vi "SetZoomMode.vi"(9 "Coords":T1, 10 "ZoomMode":refnum<vi>, 11 "XYGraph输入":refnum<vi>) -> ()   [LabVIEW 2015]
uses:
  <vilib>/Utility/miscctls.llb/LVPoint32TypeDef.ctl
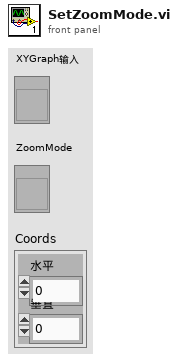
[diagram p1: front panel]
types:
  T1 = typedef "LVPoint32TypeDef.ctl" = cluster{"Horizontal":i32, "Vertical":i32}
  T2 = typedef "LVRectTypeDef.ctl" = cluster{"Left":i16, "Top":i16, "Right":i16, "Bottom":i16}
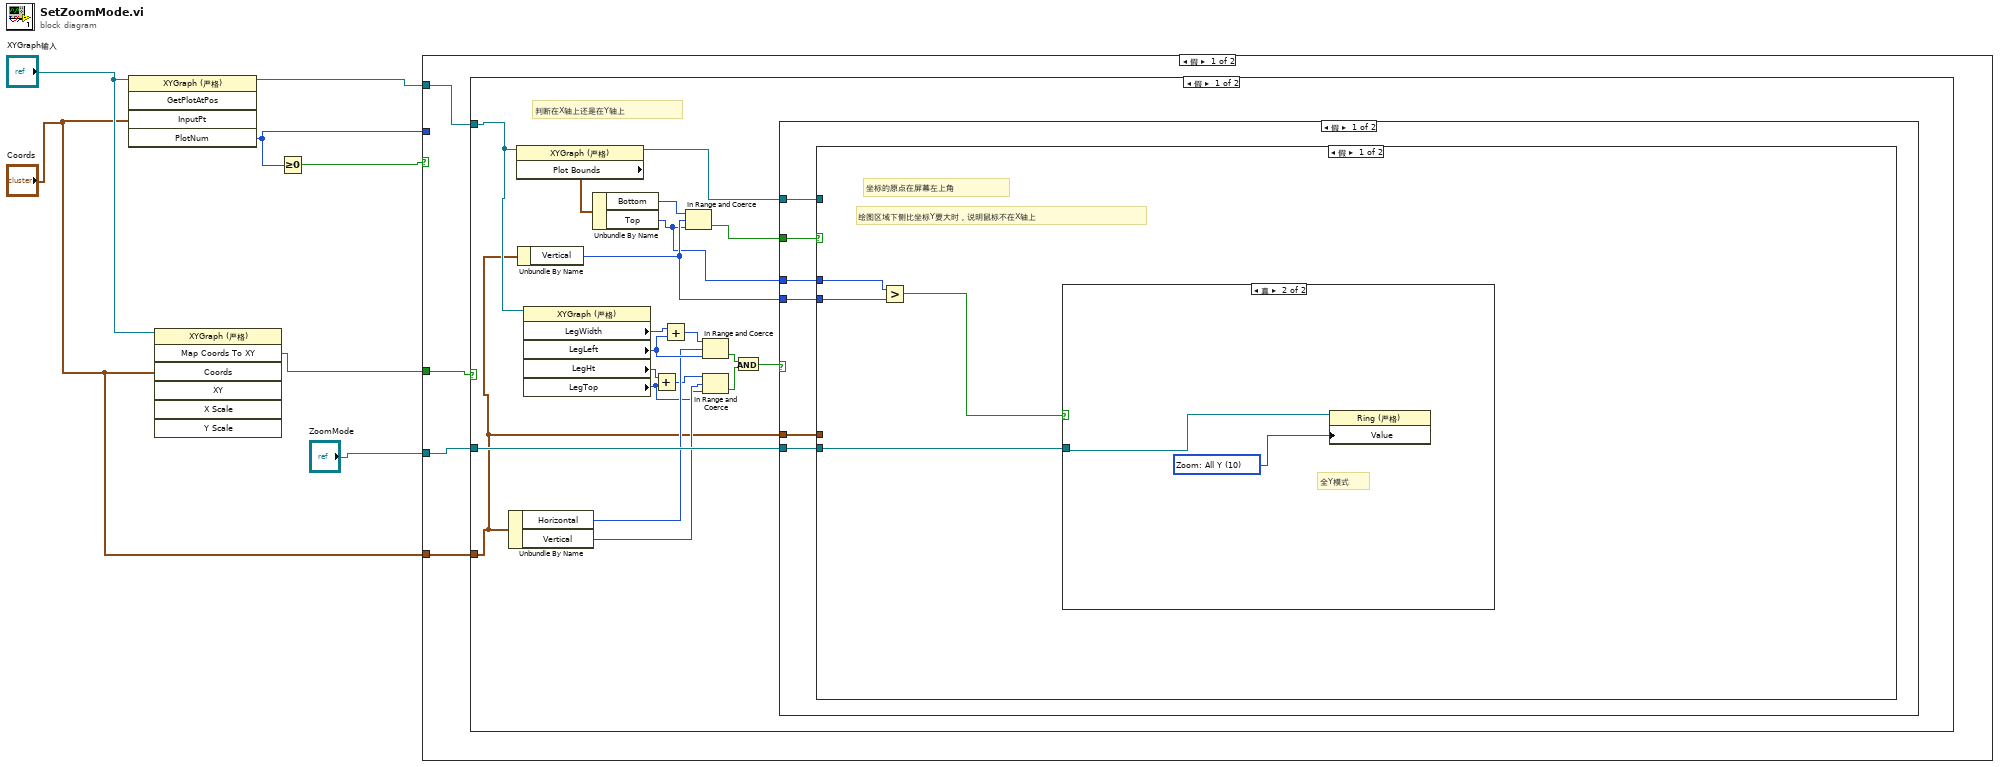
[diagram p0: block diagram]
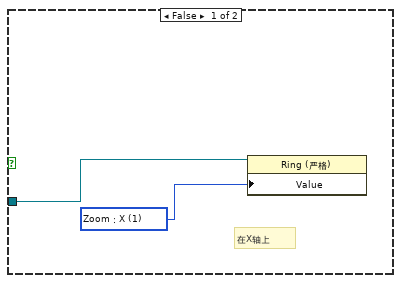
[diagram p2: hidden frame]
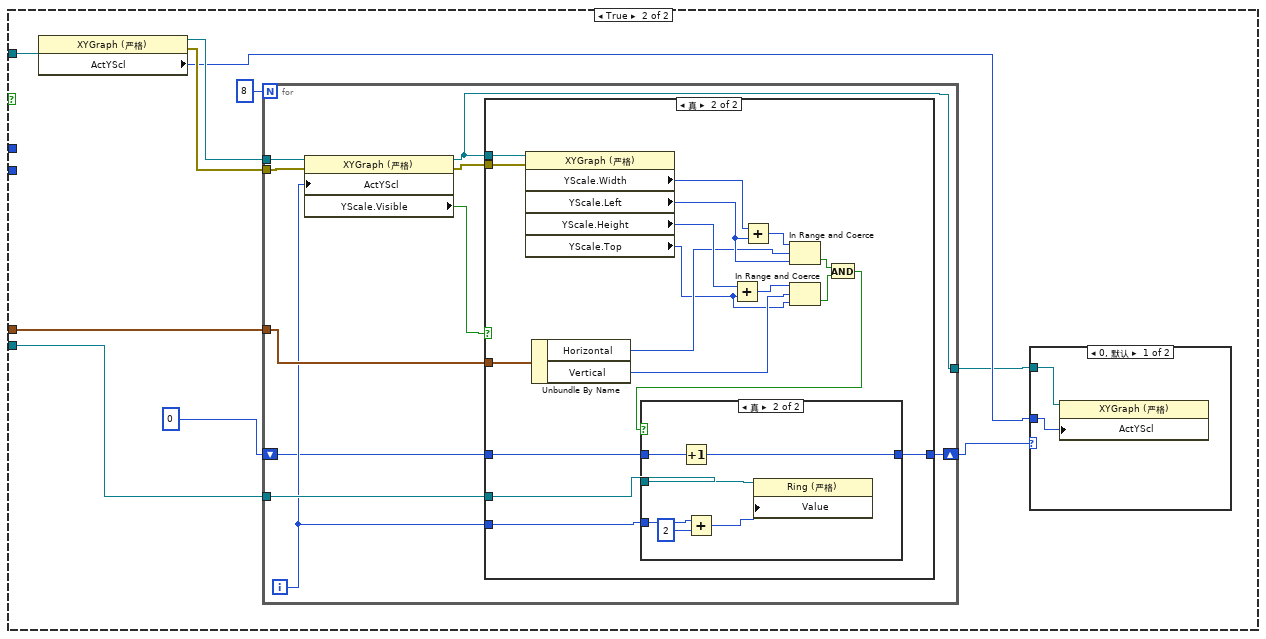
[diagram p3: hidden frame]
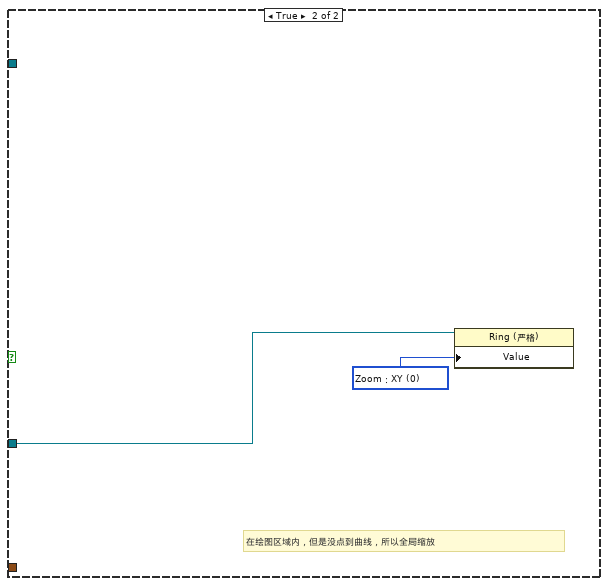
[diagram p8: hidden frame]
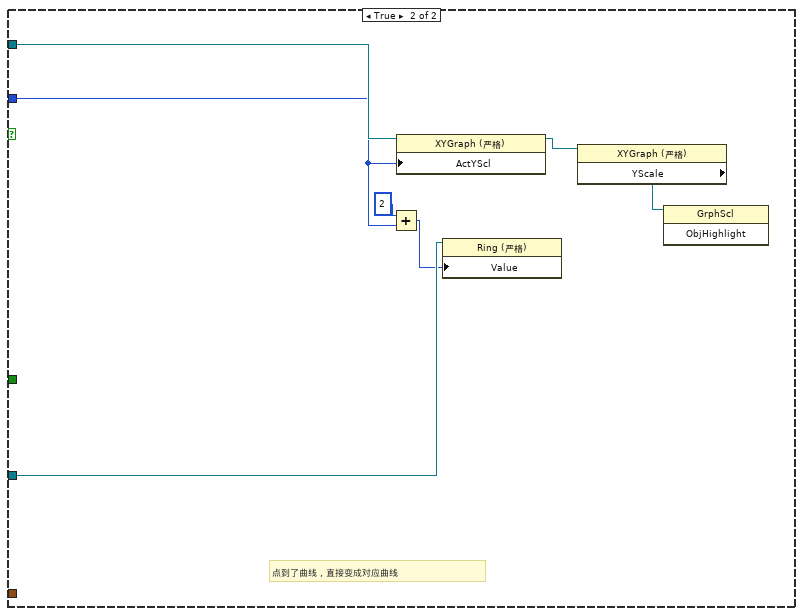
[diagram p9: hidden frame]
diagram:
  n1 = invoke class="XYGraph (严格)" method="GetPlotAtPos"(reference="XYGraph输入", "InputPt"="Coords") -> (reference out=w4:refnum<vi>, "PlotNum"=w3:i32)  [unwired: 3 in, 3 out]
  n2 = invoke class="XYGraph (严格)" method="Map Coords To XY"(reference="XYGraph输入", "Coords"="Coords") -> ("Map Coords To XY"=w6:bool)  [unwired: 5 in, 6 out]
  n3 = Greater Or Equal To 0?(x=w3) -> (x >= 0?=w2:bool)
  n4 = case shown="假" w2 {
    tunnel: w4 -> [w9 w102]
    tunnel: w3 -> [_ w99]
    tunnel: w6 -> [w11 _]
    tunnel: "ZoomMode" -> [w10 w98]
    tunnel: "Coords" -> [w8 _]
    frame False {
      n5 = case shown="假" w11 {
        tunnel: w10 -> [w31 w95]
        tunnel: w9 -> [w30 _]
        tunnel: w8 -> [w19 _]
        frame False {
          # "判断在X轴上还是在Y轴上"
          n6 = Unbundle By Name(w19) -> ("Horizontal"=w26:i32, "Vertical"=w24:i32)
          n7 = property class="XYGraph (严格)"(reference=w30) -> (reference out=w20:refnum<vi>, "Plot Bounds"=w18:T2)  [unwired: 1 in, 1 out]
          n8 = Unbundle By Name(w19) -> ("Vertical"=w13:i32)
          n9 = property class="XYGraph (严格)"(reference=w30) -> ("LegWidth"=w29:u32, "LegLeft"=w27:i32, "LegHt"=w25:u32, "LegTop"=w17:i32)  [unwired: 1 in, 2 out]
          n10 = Unbundle By Name(w18) -> ("Bottom"=w15:i16, "Top"=w12:i16)
          n11 = Add(x=w25, y=w17) -> (x+y=w16:u32)
          n12 = Add(x=w29, y=w27) -> (x+y=w28:u32)
          n13 = In Range and Coerce(upper limit=w15, x=w13, lower limit=w12) -> (In Range?=w14:bool)  [unwired: 1 out]
          n14 = In Range and Coerce(upper limit=w28, x=w26, lower limit=w27) -> (In Range?=w23:bool)  [unwired: 1 out]
          n15 = In Range and Coerce(upper limit=w16, x=w24, lower limit=w17) -> (In Range?=w22:bool)  [unwired: 1 out]
          n16 = And(x=w23, y=w22) -> (x .and. y?=w21:bool)
          n17 = case shown="假" w21 {
            tunnel: w14 -> [w37 _]
            tunnel: w31 -> [w36 _]
            tunnel: w20 -> [w35 _]
            tunnel: w19 -> [w34 _]
            tunnel: w13 -> [w33 _]
            tunnel: w12 -> [w32 _]
            frame False {
              n18 = case shown="假" w37 {
                tunnel: w36 -> [w41 w50]
                tunnel: w35 -> [_ w54]
                tunnel: w34 -> [_ w51]
                tunnel: w33 -> [w38 _]
                tunnel: w32 -> [w39 _]
                frame False {
                  # "绘图区域下侧比坐标Y要大时，说明鼠标不在X轴上"
                  # "坐标的原点在屏幕左上角"
                  n19 = Greater?(x=w39, y=w38) -> (0:w40:bool)
                  n20 = case shown="真" w40 {
                    tunnel: w41 -> [w43 w44]
                    frame False {
                      w42 = u16 1 items=["Zoom：XY", "Zoom：X", "Zoom：Y1", "Zoom：Y2", "Zoom：Y3", "Zoom：Y4", "Zoom：Y5", "Zoom：Y6", "Zoom：Y7", "Zoom：Y8", "Zoom: All Y"] ("ZoomMode")
                      # "在X轴上"
                      n21 = property class="Ring (严格)"(reference=w43, "Value"=w42) -> ()  [unwired: 1 in, 2 out]
                    }
                    frame True {
                      w45 = u16 10 items=["Zoom：XY", "Zoom：X", "Zoom：Y1", "Zoom：Y2", "Zoom：Y3", "Zoom：Y4", "Zoom：Y5", "Zoom：Y6", "Zoom：Y7", "Zoom：Y8", "Zoom: All Y"] ("ZoomMode")
                      # "全Y模式"
                      n22 = property class="Ring (严格)"(reference=w44, "Value"=w45) -> ()  [unwired: 1 in, 2 out]
                    }
                  }
                }
                frame True {
                  n23 = property class="XYGraph (严格)"(reference=w54) -> (reference out=w53:refnum<vi>, error out=w52:errorcluster, "ActYScl"=w47:i32)  [unwired: 1 in]
                  n24 = for {
                    N: 8 -> [_]
                    tunnel: w53 -> [w67]
                    tunnel: w52 -> [w65]
                    tunnel: w51 -> [w63]
                    tunnel: w50 -> [w62]
                    shift-right: [w60] -> w48
                    shift-left: 0 -> [w59]
                    tunnel: [w58] -> w46
                    i -> [w61]
                    n25 = property class="XYGraph (严格)"(reference=w67, error in=w65, "ActYScl"=w61) -> (reference out=w58:refnum<vi>, error out=w66:errorcluster, "YScale.Visible"=w64:bool)
                    n26 = case shown="真" w64 {
                      tunnel: w58 -> [_ w81]
                      tunnel: w66 -> [_ w80]
                      tunnel: w63 -> [_ w78]
                      tunnel: w62 -> [_ w74]
                      tunnel: w61 -> [_ w73]
                      tunnel: [w68 w72] -> w60
                      tunnel: w59 -> [w68 w71]
                      frame False {
                      }
                      frame True {
                        n27 = property class="XYGraph (严格)"(reference=w81, error in=w80) -> ("YScale.Width"=w83:u32, "YScale.Left"=w82:i32, "YScale.Height"=w79:u32, "YScale.Top"=w69:i32)  [unwired: 2 out]
                        n28 = Unbundle By Name(w78) -> ("Horizontal"=w77:i32, "Vertical"=w76:i32)
                        n29 = Add(x=w79, y=w69) -> (x+y=w70:u32)
                        n30 = Add(x=w83, y=w82) -> (x+y=w84:u32)
                        n31 = In Range and Coerce(upper limit=w84, x=w77, lower limit=w82) -> (In Range?=w85:bool)  [unwired: 1 out]
                        n32 = In Range and Coerce(upper limit=w70, x=w76, lower limit=w69) -> (In Range?=w86:bool)  [unwired: 1 out]
                        n33 = And(x=w85, y=w86) -> (x .and. y?=w75:bool)
                        n34 = case shown="真" w75 {
                          tunnel: w74 -> [_ w93]
                          tunnel: w73 -> [_ w92]
                          tunnel: w71 -> [w87 w89]
                          tunnel: [w87 w88] -> w72
                          frame False {
                          }
                          frame True {
                            n35 = Increment(x=w89) -> (x+1=w88:i32)
                            n36 = Add(x=w92, y=2) -> (x+y=w91:i32)
                            n37 = property class="Ring (严格)"(reference=w93, "Value"=w91) -> ()  [unwired: 1 in, 2 out]
                          }
                        }
                      }
                    }
                  }
                  n38 = case shown="0, 默认" w48 {
                    tunnel: w47 -> [w56 _]
                    tunnel: w46 -> [w57 _]
                    frame 0, Default {
                      n39 = property class="XYGraph (严格)"(reference=w57, "ActYScl"=w56) -> ()  [unwired: 1 in, 2 out]
                    }
                    frame 1 {
                    }
                  }
                }
              }
            }
            frame True {
              # "鼠标在图例上，不响应"
            }
          }
        }
        frame True {
          w94 = u16 0 items=["Zoom：XY", "Zoom：X", "Zoom：Y1", "Zoom：Y2", "Zoom：Y3", "Zoom：Y4", "Zoom：Y5", "Zoom：Y6", "Zoom：Y7", "Zoom：Y8"] ("ZoomMode")
          # "在绘图区域内，但是没点到曲线，所以全局缩放"
          n40 = property class="Ring (严格)"(reference=w95, "Value"=w94) -> ()  [unwired: 1 in, 2 out]
        }
      }
    }
    frame True {
      # "点到了曲线，直接变成对应曲线"
      n41 = Add(x=2, y=w99) -> (x+y=w97:i32)
      n42 = property class="XYGraph (严格)"(reference=w102, "ActYScl"=w99) -> (reference out=w101:refnum<vi>)  [unwired: 1 in, 1 out]
      n43 = property class="Ring (严格)"(reference=w98, "Value"=w97) -> ()  [unwired: 1 in, 2 out]
      n44 = property class="XYGraph (严格)"(reference=w101) -> ("YScale"=w100:refnum<vi>)  [unwired: 1 in, 2 out]
      n45 = invoke class="GrphScl" method="ObjHighlight"(reference=w100) -> ()  [unwired: 2 in, 3 out]
    }
  }
